vi "Write.Data.Buffer.vi"(8 "error in (no error)":errorcluster, 9 "Offset":i32, 10 "Values":dbl[](array[numeric]), 11 "Ref":refnum<data-value>) -> (0 "error out":errorcluster)   [LabVIEW 2015, in "Data Access Engine.lvlib" / "Data Access Engine.lvclass"]
uses:
  Data Access Engine.lvclass
  Access Type Classes/Write/Write.lvclass
  Access Type Classes/Write/Write.lvclass/Write.ctl
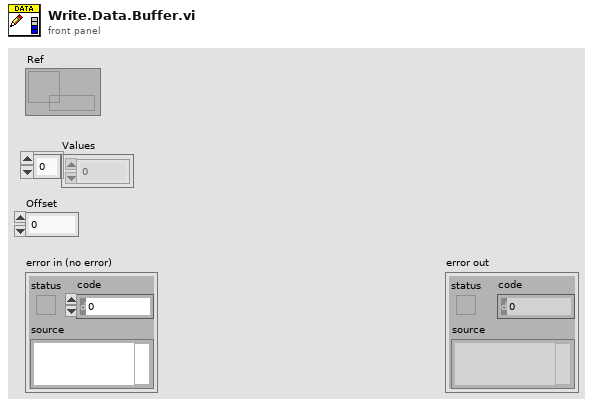
[diagram p1: front panel]
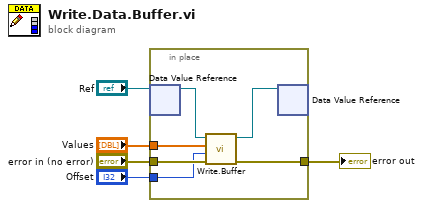
[diagram p0: block diagram]
diagram:
  n1 = in-place {
    in-place-border: "error in (no error)" -> [w11]
    in-place-border: [w10] -> w4
    in-place-border: "Values" -> [w7]
    in-place-border: "Offset" -> [w6]
    n2 = in-place-dvr #1("Ref") -> (w9:refnum<class "Write.lvclass">)  [unwired: 1 out]
    n3 = call "Write.Buffer.vi"("error in (no error)"=w11, "Offset"=w6, "Values"=w7, "Write in"=w9) -> ("error out"=w10:errorcluster, "Write out"=w8:refnum<class "Write.lvclass">)  [unwired: 6 in]
    n4 = in-place-dvr #1(w8) -> ()  [unwired: 2 out]
  }
  "error out" <- w4
